vi "GetCoeffsAndComp.vi"(8 "Apply Phase Correction?":bool=TRUE, 10 "mutedData":dbl[](array[numeric]), 11 "TubingCorrectionFile":path) -> (2 "boostedData":dbl[](array[numeric]))   [LabVIEW 2013]
uses:
  Globals/Meas_global.vi
panel:
  in  "Refresh Button":bool
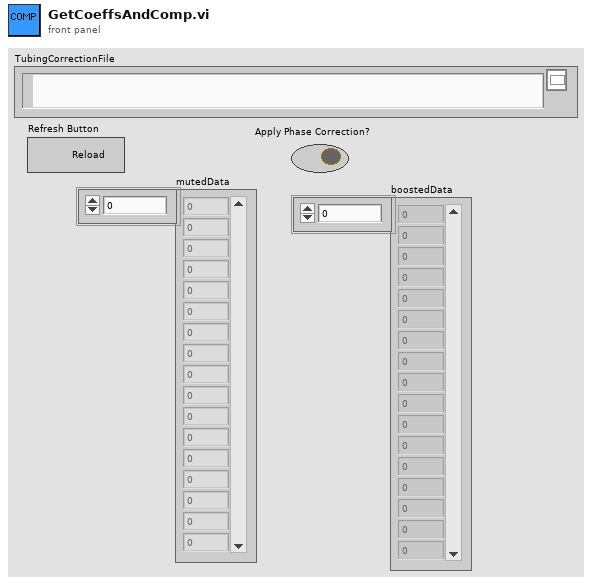
[diagram p1: front panel]
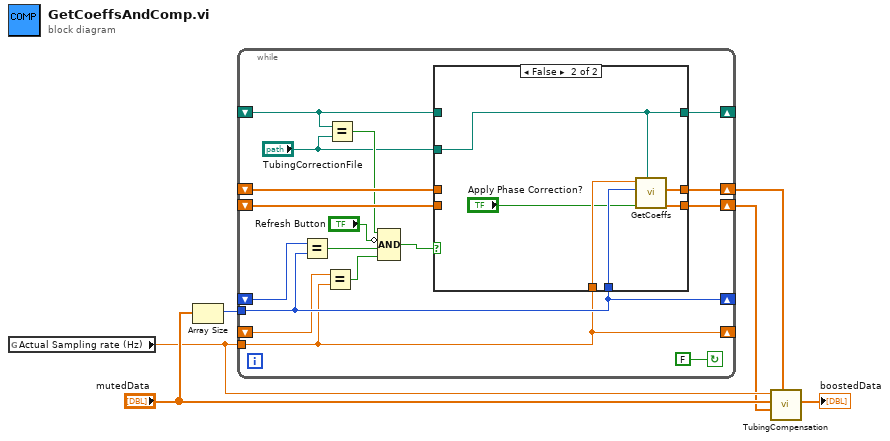
[diagram p0: block diagram]
diagram:
  n1 = global read "Meas_global.vi" "Actual Sampling rate (Hz)"() -> (w3:dbl)
  n2 = Array Size(array="mutedData") -> (size(s)=w5:i32)
  n3 = while {
    shift-right: [w22] -> w2
    shift-left: _ -> [w23]
    shift-right: [w19] -> _
    shift-left: _ -> [w20]
    shift-right: [w17] -> _
    shift-left: _ -> [w18]
    tunnel: w5 -> [w19]
    tunnel: w3 -> [w17]
    shift-right: [w14] -> _
    shift-left: _ -> [w7]
    shift-right: [w13] -> w1
    shift-left: _ -> [w12]
    stop <- FALSE continue-if-true
    n4 = Equal?(x=w20, y=w19) -> (x = y?=w15:bool)
    n5 = Equal?(x=w18, y=w17) -> (x = y?=w16:bool)
    n6 = Equal?(x=w7, y="TubingCorrectionFile") -> (x = y?=w9:bool)
    n7 = Compound Arithmetic op=AND(w9, invert "Refresh Button", w15, w16) -> (w11:bool)
    n8 = case shown="False" w11 {
      tunnel: [w26 w32] -> w22
      tunnel: w23 -> [w26 _]
      tunnel: w17 -> [_ w31]
      tunnel: w19 -> [_ w30]
      tunnel: [w25 w27] -> w14
      tunnel: w7 -> [w25 _]
      tunnel: [w24 w28] -> w13
      tunnel: w12 -> [w24 _]
      tunnel: "TubingCorrectionFile" -> [_ w27]
      frame True {
      }
      frame False {
        n9 = call "GetCoeffs.vi"("PathToFile"=w27, "Apply Phase Correction?"="Apply Phase Correction?", "SignalLength"=w30, "fs (Hz)"=w31) -> ("NyquistLimitedPhase"=w28:dbl[], "NyquistLimitedCoefficients"=w32:dbl[])  [unwired: 6 in]
      }
    }
  }
  n10 = call "TubingCompensation.vi"("NyquistLimitedCoefficients"=w2, "NyquistLimitedPhase"=w1, "mutedData"="mutedData", "SamplingFreq"=w3) -> ("boostedData"=→"boostedData":dbl[])  [unwired: 7 in]
